vi "SumList.vi"(8 "error in (no error)":errorcluster) -> (0 "error out":errorcluster, 3 "SumList":string[](array[string]))   [LabVIEW 2014]
uses:
  typedefs/ePathsAction.ctl
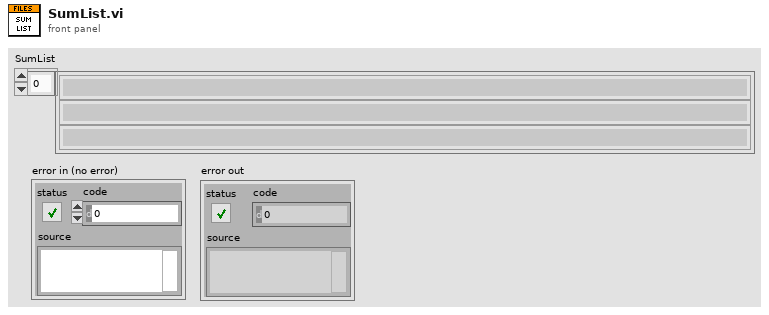
[diagram p1: front panel]
types:
  T1 = typedef "ePathsAction.ctl" = enum16{"Set", "Get", "Load", "Save", "Default", "Exit"}
  T2 = typedef "Paths.ctl" = cluster{"BasePath":path, "FlukePath":path, "LastFlukePath":path, "NISTPath":path, "LastNISTPath":path, "ResultsPath":path}
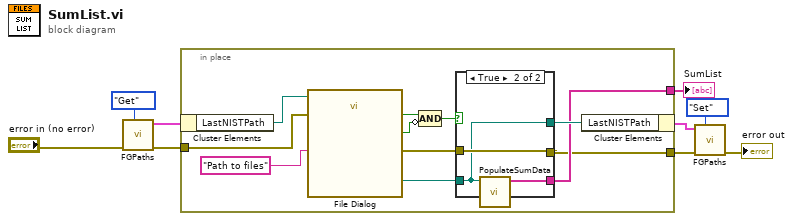
[diagram p0: block diagram]
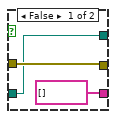
[diagram p2: hidden frame]
diagram:
  n1 = call "FGPaths.vi"("ePathsAction"=ePathsAction."Get", "error in (no error)"="error in (no error)") -> ("error out"=w7:errorcluster, "PathsOut"=w6:T2)  [unwired: 8 in]
  n2 = in-place {
    in-place-border: w7 -> [w19]
    in-place-border: [w11] -> w2
    in-place-border: [w10] -> w8
    n3 = in-place-cluster #1(w6) -> ("LastNISTPath"=w20:path)
    n4 = call "File Dialog"("start path"=w20, "prompt"="Path to files", "error in"=w19) -> ("selected path"=w13:path, "exists"=w17:bool, "cancelled"=w16:bool, "error out"=w14:errorcluster)  [unwired: 9 in]
    n5 = Compound Arithmetic op=AND(w17, invert w16) -> (w15:bool)
    n6 = case shown="True" w15 {
      tunnel: [w22 w26] -> w10
      tunnel: w14 -> [w22 w26]
      tunnel: w13 -> [w21 w25]
      tunnel: [w21 w25] -> w12
      tunnel: [string[] [] ("Array") w24] -> w11
      frame False {
      }
      frame True {
        n7 = call "PopulateSumData.vi"("Path"=w25) -> ("Array"=w24:string[])  [unwired: 10 in]
      }
    }
    n8 = in-place-cluster #1("LastNISTPath"=w12) -> (w9:T2)
  }
  "SumList" <- w2
  n9 = call "FGPaths.vi"("ePathsAction"=ePathsAction."Set", "error in (no error)"=w8, "PathsIn"=w9) -> ("error out"=→"error out":errorcluster)  [unwired: 7 in, 1 out]
